vi "ErrorCatcher.vi"(8 "error in (no error)":errorcluster, 10 "Test Daten":T1={"commandlist"="", "line"=0, "last response"="", "timeout"=0, "wait"=0, "erfolgreich"=FALSE, "next state"=enum."init", "Zustand"=enum."starting", "manual Test"=FALSE}, 11 "Tektronix RSA5106A in":refnum<class "Tektronix RSA5106A.lvclass">) -> (0 "error out":errorcluster, 3 "Tektronix RSA5106A out":refnum<class "Tektronix RSA5106A.lvclass">)   [LabVIEW 2013, in "Tektronix RSA5106A.lvclass"]
uses:
  Tektronix RSA5106A.lvclass
  Main/controls/TestData.ctl
  Main/controls/TestStates.ctl
  Main/controls/generalTestStates.ctl
  <vilib>/regexp/Match Regular Expression.xnode
  lib/EMV-Test.lvlib
panel:
  out "VISA Refnum out":refnum<visa-resource-name>
  out "error code":i32
  out "error msg":string
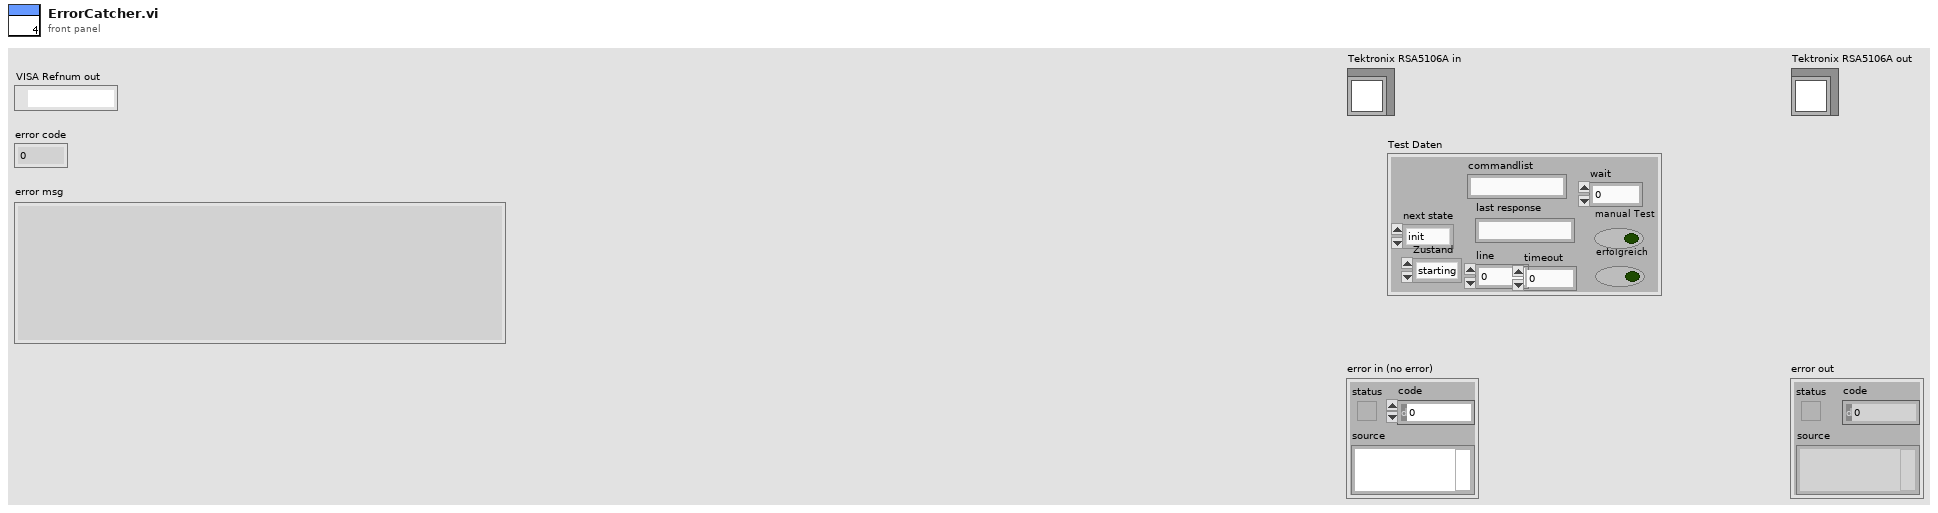
[diagram p1: front panel]
types:
  T1 = typedef "EMV-Test.lvlib/TestData.ctl" = cluster{"commandlist":string, "line":i32, "last response":string, "timeout":i32, "wait":u32, "erfolgreich":bool, "next state":T2, "Zustand":T3, "manual Test":bool}
  T2 = typedef "EMV-Test.lvlib/TestStates.ctl" = enum16{"event loop", "save Test", "Custom Action 1", "Custom Action 2", "pause", "vorgefertigter Test", "manueller Test", "respond to response", "error", "init", "start Test", "evaluate line", "wait for Response", "wait", "catch error", "close Connection", "end"}
  T3 = typedef "generalTestStates.ctl" = enum16{"paused", "starting", "waiting", "running", "finished"}
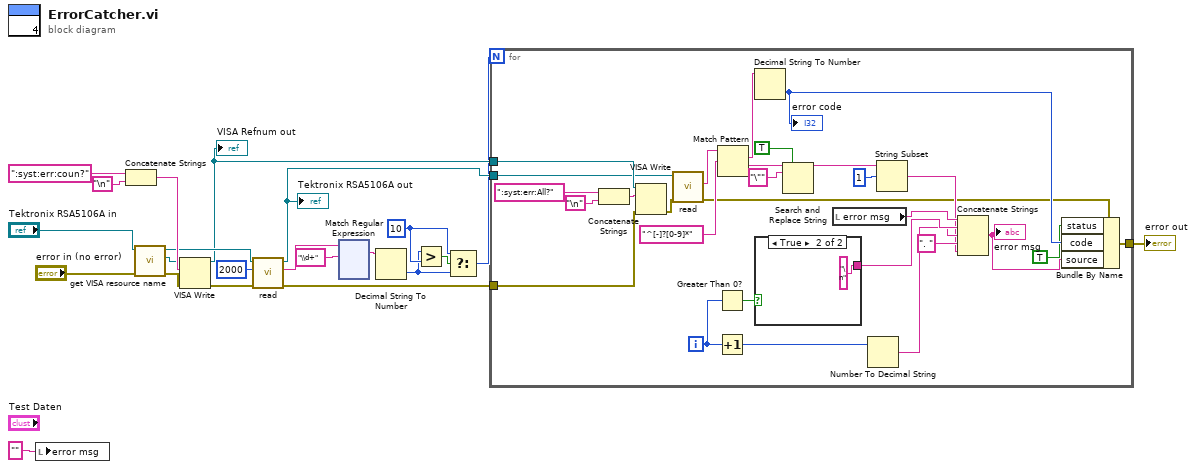
[diagram p0: block diagram]
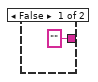
[diagram p2: hidden frame]
diagram:
  w3 = 10 ("y")
  n1 = local write "error msg"("" ("error msg")) -> ()
  n2 = Concatenate Strings(":syst:err:coun?" ("string"), "\n") -> (w17:string)
  n3 = call-dynamic "get VISA resource name.vi"("error in (no error)"="error in (no error)", "DeviceInterface (Eingang)"="Tektronix RSA5106A in") -> ("error out"=w13:errorcluster, "VISA resource name"=w12:refnum<visa-resource-name>, "DeviceInterface (Ausgang)"=w11:refnum<class "Tektronix RSA5106A.lvclass">)  [unwired: 7 in]
  n4 = VISA Write(VISA resource name=w12, write buffer=w17, error in (no error)=w13) -> (VISA resource name out=w6:refnum<visa-resource-name>, error out=w8:errorcluster)  [unwired: 1 out]
  "VISA Refnum out" <- w6
  n5 = call-dynamic "read.vi"("error in (no error)"=w8, "timeout (ms)"=2000, "Tektronix RSA5106A in"=w11) -> ("error out"=w9:errorcluster, "Return String"=w10:string, "Tektronix RSA5106A out"=w5:refnum<class "Tektronix RSA5106A.lvclass">)  [unwired: 6 in]
  "Tektronix RSA5106A out" <- w5
  n6 = xnode "Match Regular Expression"("input string"=w10, "regular expression"="\\d+") -> ("whole match"=w19:string)  [unwired: 4 in, 4 out]
  n7 = Decimal String To Number(string=w19) -> (number=w2:i32)  [unwired: 2 in, 1 out]
  n8 = Greater?(x=w2, y=w3) -> (0:w4:bool)
  n9 = Select(t=w3, s=w4, f=w2) -> (s? t:f=w1:i32)
  n10 = for {
    N: w1 -> [_]
    tunnel: [w39] -> w14
    tunnel: w9 -> [w28]
    tunnel: w6 -> [w47]
    tunnel: w5 -> [w30]
    i -> [w41]
    n11 = Concatenate Strings(":syst:err:All?" ("string"), "\n") -> (w48:string)
    n12 = VISA Write(VISA resource name=w47, write buffer=w48, error in (no error)=w28) -> (error out=w31:errorcluster)  [unwired: 2 out]
    n13 = call-dynamic "read.vi"("error in (no error)"=w31, "Tektronix RSA5106A in"=w30) -> ("error out"=w27:errorcluster, "Return String"=w29:string)  [unwired: 7 in, 1 out]
    n14 = Greater Than 0?(x=w41) -> (x > 0?=w42:bool)
    n15 = Increment(x=w41) -> (x+1=w43:i32)
    n16 = Match Pattern(string=w29, regular expression="^[-]?[0-9]*") -> (match substring=w46:string, after substring=w24:string)  [unwired: 1 in, 2 out]
    n17 = Decimal String To Number(string=w46) -> (number=w37:i32)  [unwired: 2 in, 1 out]
    "error code" <- w37
    n18 = case shown="True" w42 {
      tunnel: ["" ("string") "\n" ("string")] -> w40
      frame False {
      }
      frame True {
      }
    }
    n19 = Search and Replace String(replace all?=TRUE ("replace all? (F)"), input string=w24, search string="\"") -> (result string=w23:string)  [unwired: 1 in, 7 out]
    n20 = local read "error msg"() -> (w35:string)
    n21 = Number To Decimal String(number=w43) -> (decimal integer string=w34:string)  [unwired: 1 in]
    n22 = String Subset(string=w23, offset (0)=1) -> (substring=w32:string)  [unwired: 1 in]
    n23 = Concatenate Strings(w35, w40, w34, ". " ("string"), w32) -> (w38:string)
    "error msg" <- w38
    n24 = Bundle By Name(cluster=w27, "status"=TRUE, "code"=w37, "source"=w38) -> (w39:errorcluster)
  }
  "error out" <- w14
